vi "Set Open List.vi"(10 "Priority Queue.lvclass":refnum<class "NI_Robotics_Priority Queue.lvclass">, 11 "AD* in":refnum<class "NI_Robotics_AnytimeDStar.lvclass">) -> (3 "AD* out":refnum<class "NI_Robotics_AnytimeDStar.lvclass">)   [LabVIEW 2017, in "NI_Robotics_AnytimeDStar.lvclass"]
uses:
  <vilib>/robotics/Navigation/Anytime D Star/NI_Robotics_AnytimeDStar.lvclass
  <vilib>/robotics/Navigation/shared/Priority Queue/NI_Robotics_Priority Queue.lvclass
  <vilib>/robotics/Navigation/Anytime D Star/NI_Robotics_AnytimeDStar.lvclass/NI_Robotics_AnytimeDStar.ctl
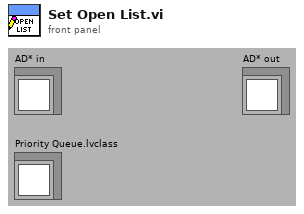
[diagram p1: front panel]
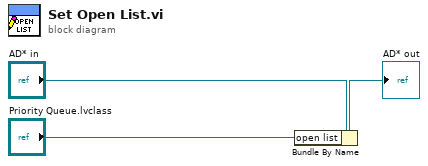
[diagram p0: block diagram]
diagram:
  n1 = Bundle By Name(cluster="AD* in", "open list"="Priority Queue.lvclass") -> (→"AD* out":refnum<class "NI_Robotics_AnytimeDStar.lvclass">)
